vi "_080.vi"() -> ()   [LabVIEW 2024]
panel:
  out "initialized array":i32[](array[numeric])
  out "Array 2":i32[](array[numeric])
  out "Array":i32[](array[numeric])
  # "Fundamentals :"
  # "9~>After running this VI,what is the value displayed in the o/p ?"
  # "Nrml Approach :"
  # "Dfrnt Approach :"
  # "( Work flow )"
  # "The working of intitialize array is we have to print the element particular times ,9 is the element and 3 is the dimension size(how many times have to print the nine & then the loop will run 3 times & the iteration will val is  2 , 1st the 9 will stored in replace array subsetb & simultaneously the  zero'the iteration will be in false condition and  1st iteration 1 will incremented to 2 & then pushed to replace array subset & then 2nd iteration incremented to 3 & then pushed to replace array subset.Finallay the output 9,2,3"
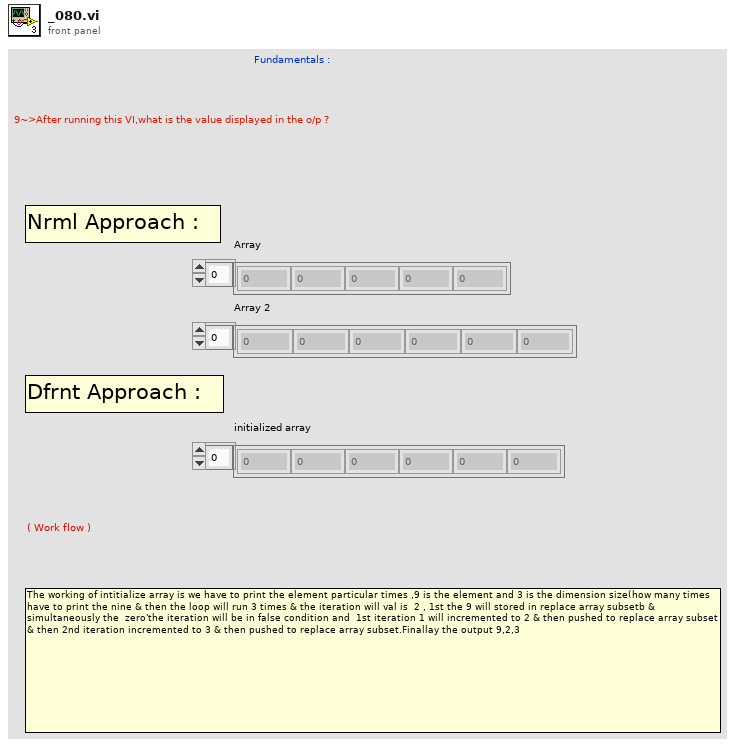
[diagram p1: front panel]
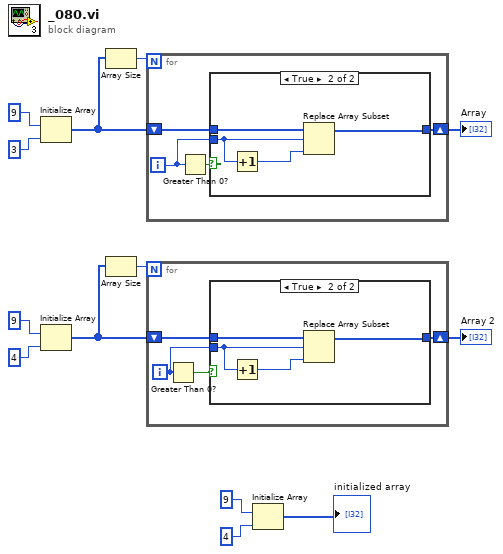
[diagram p0: block diagram]
diagram:
  n1 = Initialize Array "Initialize Array"(9, 3) -> (w12:i32[])
  n2 = Initialize Array "Initialize Array"(9, 4) -> (w5:i32[])
  n3 = Array Size(array=w12) -> (size(s)=w11:i32)
  n4 = Array Size(array=w5) -> (size(s)=w6:i32)
  n5 = for {
    N: w11 -> [_]
    shift-right: [w16] -> w10
    shift-left: w12 -> [w17]
    i -> [w14]
    n6 = Greater Than 0?(x=w14) -> (x > 0?=w15:bool)
    n7 = case shown="True" w15 {
      tunnel: w17 -> [w18 w22]
      tunnel: [w18 w21] -> w16
      tunnel: w14 -> [_ w20]
      frame False {
      }
      frame True {
        n8 = Increment(x=w20) -> (x+1=w19:i32)
        n9 = Replace Array Subset "Replace Array Subset"(array=w22, new element=w19, index=w20) -> (w21:i32[])
      }
    }
  }
  "Array" <- w10
  n10 = for {
    N: w6 -> [_]
    shift-right: [w25] -> w7
    shift-left: w5 -> [w26]
    i -> [w23]
    n11 = Greater Than 0?(x=w23) -> (x > 0?=w24:bool)
    n12 = case shown="True" w24 {
      tunnel: w26 -> [w27 w31]
      tunnel: [w27 w30] -> w25
      tunnel: w23 -> [_ w29]
      frame False {
      }
      frame True {
        n13 = Increment(x=w29) -> (x+1=w28:i32)
        n14 = Replace Array Subset "Replace Array Subset"(array=w31, new element=w28, index=w29) -> (w30:i32[])
      }
    }
  }
  "Array 2" <- w7
  n15 = Initialize Array "Initialize Array"(9, 4) -> (→"initialized array":i32[])
